vi "PowerMeterCheck.vi"(1 "错误输入（无错误）":errorcluster) -> (2 "通信正常？":bool, 4 "错误输出":errorcluster)   [LabVIEW 2018]
panel:
  out "字符串":string="功率计表头"
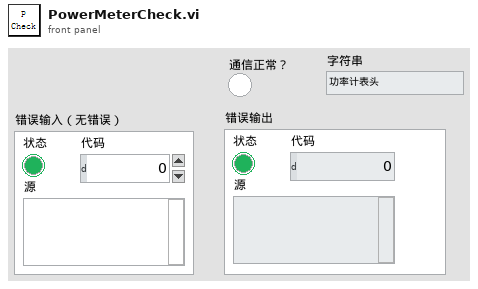
[diagram p1: front panel]
types:
  T1 = enum16{"Standard", "Buffered", "CRLF", "Immediate"}
  T2 = typedef "IMAQ Image.ctl" = refnum<image>
  T3 = cluster{"示波器":cluster{"Channel (0:Channel 1)":enum16{"Channel 1", "Channel 2", "Channel 3", "Channel 4"}, "电压范围":dbl, "触发电压":dbl, "时间范围":dbl, " 示波器VISA":refnum<visa-resource-name>, "电压范围 标签":u64, "时间范围 标签":u64}, "光谱仪":cluster{"Channel (0:Channel 1)":enum16{"Channel 1", "Channel 2", "Channel 3", "Channel 4"}, "电压范围":u64, "触发电压":u64, "时间范围":u64}, " 近场相机":cluster{"曝光时间":i32, "模拟增益":i32, "控制套接字":i32, "IP 地址":string, " 采集套接字":i32, "  版本号":i32, "ImageData":T2, "  增益最大":i32, "  增益最小":i32, " 曝光最大":i32, " 曝光最小":i32, " 帧速":i32, " 同步切换":i32, "  曝光缩放":i32}, " 偏振仪":cluster{"电压范围":u64, "触发电压":u64, "时间范围":u64, "波长范围":enum16{"可见光 400-700nm", "近红外 700-1100nm"}}, " 功率计":cluster{"通道":enum16{"Channel 1", "Channel 2"}, "工作波长":u32, "单位":u64, "时间范围":u64, "IP地址":string, "端口":u32}, "能量计":cluster{"通道":enum16{"Channel 1", "Channel 2"}, "工作波长":u32, "单位":u64, "时间范围":u64, "IP地址":string, "端口":u32, "能量计量程":enum16{"200uJ", "20uJ", "2uJ", "200nJ"}}, "电机":cluster{"Channel (0:Channel 1)":enum16{"Channel 1", "Channel 2", "Channel 3", "Channel 4"}, "电压范围":u64, "触发电压":u64, "时间范围":u64}, " 远场相机":cluster{"曝光时间":i32, "模拟增益":i32, "控制套接字":i32, "IP 地址":string, " 采集套接字":i32, "  版本号":i32, "ImageData":T2, "  增益最大":i32, "  增益最小":i32, " 曝光最大":i32, " 曝光最小":i32, " 帧速":i32, " 同步切换":i32, "  曝光缩放":i32}}
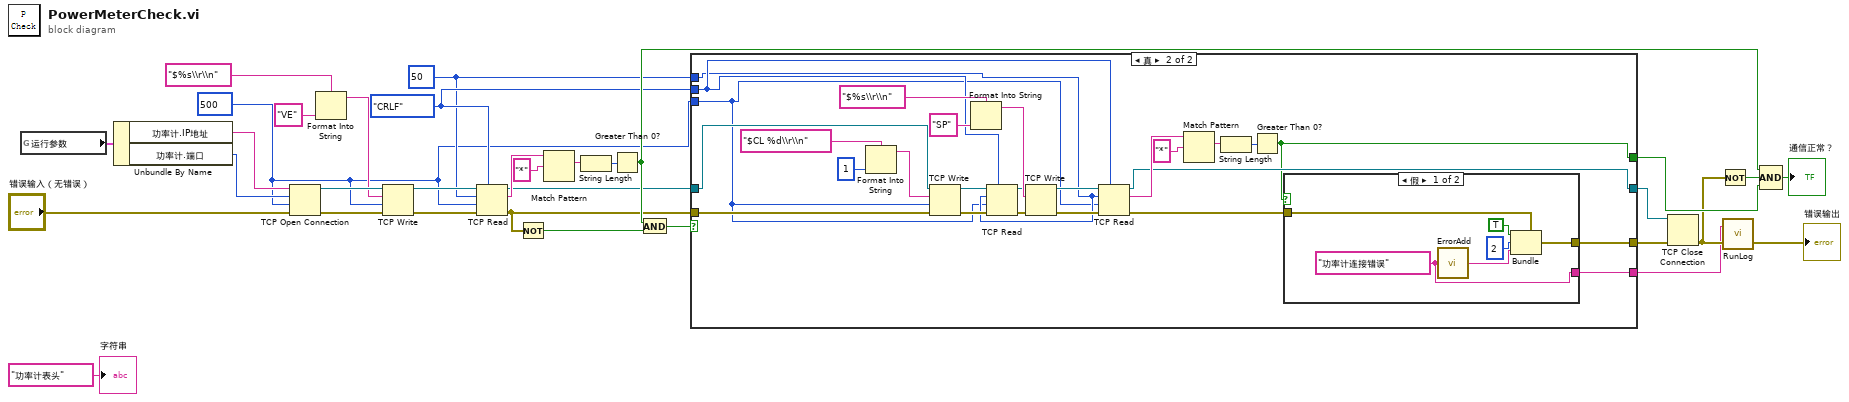
[diagram p0: block diagram]
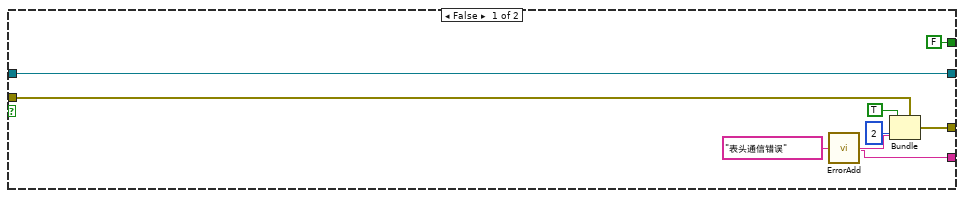
[diagram p2: hidden frame]
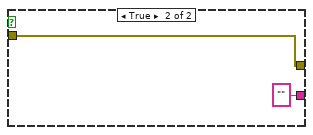
[diagram p3: hidden frame]
diagram:
  w10 = T1."CRLF" ("模式（标准）")
  w9 = 50 ("读取的字节")
  w8 = 500 ("超时毫秒(60000)")
  n1 = global read "参数.vi" "运行参数"() -> (w32:T3)
  n2 = Unbundle By Name(w32) -> ("功率计.IP地址"=w31:string, "功率计.端口"=w30:u32)
  n3 = TCP Open Connection(address=w31, remote port or service name=w30, timeout ms (60000)=w8, error in (no error)="错误输入（无错误）") -> (connection ID=w29:refnum<k5>, error out=w28:errorcluster)  [unwired: 1 in]
  n4 = Format Into String(format string="$%s\\r\\n" ("格式字符串"), "VE" ("数据输入")) -> (resulting string=w23:string)  [unwired: 2 in, 1 out]
  n5 = TCP Write(connection ID=w29, data in=w23, error in (no error)=w28, 9:w8) -> (connection ID out=w27:refnum<k5>, error out=w26:errorcluster)  [unwired: 1 out]
  n6 = TCP Read(connection ID=w27, bytes to read=w9, error in (no error)=w26, 7:w10, 9:w8) -> (connection ID out=w7:refnum<k5>, data out=w22:string, error out=w13:errorcluster)
  n7 = Not(x=w13) -> (.not. x?=w12:bool)
  n8 = Match Pattern(string=w22, regular expression="*" ("正则表达式")) -> (match substring=w20:string)  [unwired: 1 in, 3 out]
  n9 = String Length(string=w20) -> (length=w19:i32)
  n10 = Greater Than 0?(x=w19) -> (x > 0?=w14:bool)
  n11 = And(x=w14, y=w12) -> (x .and. y?=w11:bool)
  n12 = case shown="真" w11 {
    tunnel: [w38 w58] -> w4
    tunnel: [w36 w57] -> w1
    tunnel: w13 -> [w35 w43]
    tunnel: w10 -> [_ w46]
    tunnel: w8 -> [_ w41]
    tunnel: w9 -> [_ w42]
    tunnel: w7 -> [w33 w50]
    tunnel: [FALSE w56] -> w6
    tunnel: [w33 w60] -> w5
    frame False {
      w36 = "表头通信错误" ("source")
      n13 = call "ErrorAdd.vi"("source"=w36) -> ("Errorout Souce"=w37:string)
      n14 = Bundle(cluster=w35, "status"=TRUE, "code"=2, "source"=w37) -> (w38:errorcluster)
    }
    frame True {
      n15 = Format Into String(format string="$CL %d\\r\\n" ("格式字符串"), 1 ("输入 1")) -> (resulting string=w49:string)  [unwired: 2 in, 1 out]
      n16 = TCP Write(connection ID=w50, data in=w49, error in (no error)=w43, 9:w41) -> (connection ID out=w48:refnum<k5>, error out=w47:errorcluster)  [unwired: 1 out]
      n17 = Format Into String(format string="$%s\\r\\n" ("格式字符串"), "SP" ("数据输入")) -> (resulting string=w55:string)  [unwired: 2 in, 1 out]
      n18 = TCP Read(connection ID=w48, bytes to read=w42, error in (no error)=w47, 7:w46, 9:w41) -> (connection ID out=w45:refnum<k5>, error out=w44:errorcluster)  [unwired: 1 out]
      n19 = TCP Write(connection ID=w45, data in=w55, error in (no error)=w44) -> (connection ID out=w62:refnum<k5>, error out=w66:errorcluster)  [unwired: 1 in, 1 out]
      n20 = TCP Read(connection ID=w62, bytes to read=w42, error in (no error)=w66, 7:w46, 9:w41) -> (connection ID out=w60:refnum<k5>, data out=w65:string, error out=w59:errorcluster)
      n21 = Match Pattern(string=w65, regular expression="*" ("正则表达式")) -> (match substring=w63:string)  [unwired: 1 in, 3 out]
      n22 = String Length(string=w63) -> (length=w64:i32)
      n23 = Greater Than 0?(x=w64) -> (x > 0?=w56:bool)
      n24 = case shown="假" w56 {
        tunnel: w59 -> [w69 w74]
        tunnel: [w68 w74] -> w58
        tunnel: [w67 ""] -> w57
        frame False {
          w67 = "功率计连接错误" ("source")
          n25 = call "ErrorAdd.vi"("source"=w67) -> ("Errorout Souce"=w70:string)
          n26 = Bundle(cluster=w69, "status"=TRUE, "code"=2, "source"=w70) -> (w68:errorcluster)
        }
        frame True {
        }
      }
    }
  }
  n27 = TCP Close Connection(connection ID=w5, error in (no error)=w4) -> (error out=w3:errorcluster)  [unwired: 1 in, 1 out]
  n28 = Not(x=w3) -> (.not. x?=w16:bool)
  n29 = call "RunLog.vi"("error in"=w3, "Message"=w1) -> ("error out"=→"错误输出":errorcluster)  [unwired: 1 in]
  n30 = Compound Arithmetic op=AND ("复合运算")(w14, w16, w6) -> (→"通信正常？":bool)
  "字符串" <- "功率计表头"
